vi "Ad-Hoc.vi"(7 "Minutes to wait":u32, 8 "error in":errorcluster, 11 "Ad-Hoc Installers":T1 {"MachineName" items=["Machine-06", "Machine-01", "Machine-02", "Machine-03", "Machine-04"]}) -> (0 "error Out":errorcluster, 3 "Array":path[](array[path]))   [LabVIEW 2013]
uses:
  MachineNames.ctl
  ControlAd-Hoc.ctl
  <vilib>/Utility/config.llb/Read Key (String).vi
  <vilib>/Utility/config.llb/NI_LVConfig.lvlib
panel:
  out "Ring 2":T2=3 items=["Machine-01", "Machine-02", "Machine-03", "Machine-04"]
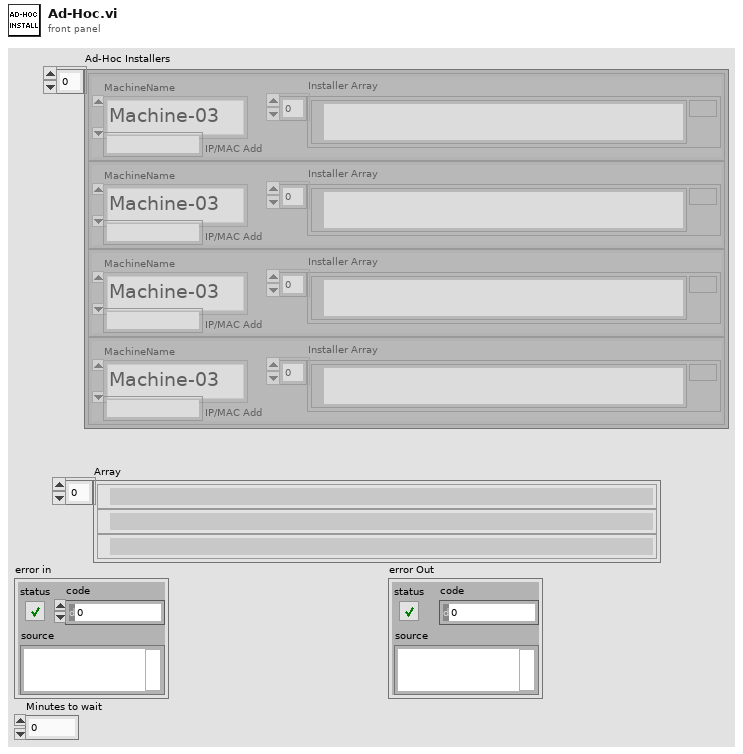
[diagram p1: front panel]
types:
  T1 = typedef "ControlAd-Hoc.ctl" = cluster{"Installer Array":path[], "MachineName":T2, "IP/MAC Add":string}[]
  T2 = typedef "MachineNames.ctl" = u16
  T3 = typedef "NI_LVConfig.lvlib/Config Data RefNum.ctl" = refnum<k1>
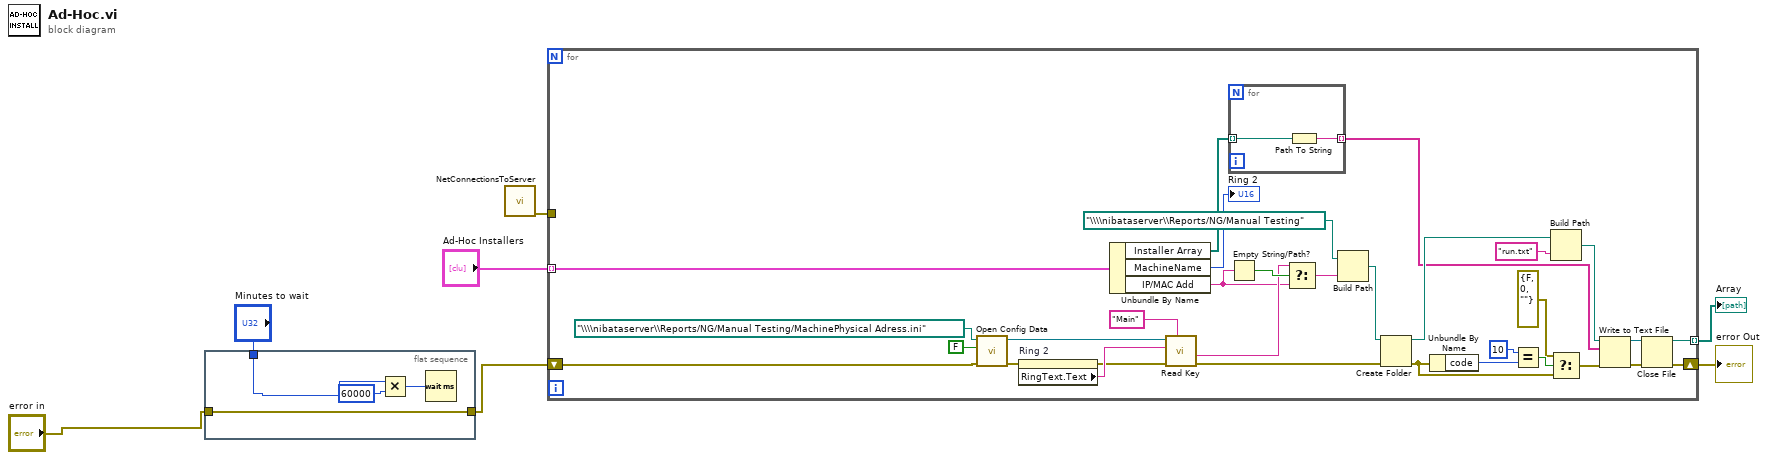
[diagram p0: block diagram]
diagram:
  n1 = flat-sequence {
    tunnel: "error in" -> [w11]
    tunnel: [w11] -> w2
    tunnel: "Minutes to wait" -> [w8]
    frame #0 {
      n2 = Multiply(x=w8, y=u32 60000) -> (x*y=w10:u32)
      n3 = Wait (ms)(milliseconds to wait=w10) -> ()  [unwired: 1 out]
    }
  }
  n4 = call "NetConnectionsToServer.vi"() -> ("error out"=w4:errorcluster)  [unwired: 11 in]
  n5 = for {
    tunnel: "Ad-Hoc Installers" -> [w43] mode=indexing
    tunnel: [w35] -> w7 mode=indexing
    shift-right: [w25] -> w5
    shift-left: w2 -> [w24]
    tunnel: w4 -> [_]
    n6 = call <vilib>:"Open Config Data.vi"("error in (no error)"=w24, "create file if necessary (T)"=FALSE, "configuration file path"=path "\\\\nibataserver\\Reports/NG/Manual Testing/MachinePhysical Adress.ini") -> ("error out"=w27:errorcluster, "refnum"=w31:T3)  [unwired: 6 in, 1 out]
    n7 = property on="Ring 2" class="Ring (strict)"(error in=w27) -> (error out=w28:errorcluster, "RingText.Text"=w29:string)  [unwired: 1 in, 1 out]
    n8 = Unbundle By Name(w43) -> ("Installer Array"=w42:path[], "MachineName"=→"Ring 2":T2, "IP/MAC Add"=w13:string)
    n9 = call-poly <vilib>:"Read Key.vi"("section"="Main", "error in (no error)"=w28, "key"=w29, "refnum"=w31) -> ("error out"=w16:errorcluster, "value"=w14:string)  [unwired: 4 in, 2 out]
    n10 = for {
      tunnel: w42 -> [w45] mode=indexing
      tunnel: [w44] -> w34 mode=indexing
      n11 = Path To String(path=w45) -> (string=w44:string)
    }
    n12 = Empty String/Path?(string/path=w13) -> (empty?=w15:bool)
    n13 = Select(t=w14, s=w15, f=w13) -> (s? t:f=w12:string)
    n14 = Build Path(base path=path "\\\\nibataserver\\Reports/NG/Manual Testing", name or relative path=w12) -> (appended path=w38:path)
    n15 = Create Folder(path (use dialog)=w38, error in=w16) -> (created path=w37:path, error out=w19:errorcluster)  [unwired: 1 in, 1 out]
    n16 = Unbundle By Name(w19) -> ("code"=w23:i32)
    n17 = Equal?(x=10, y=w23) -> (x = y?=w21:bool)
    n18 = Build Path(base path=w37, name or relative path="run.txt") -> (appended path=w40:path)
    n19 = Select(t=errorcluster {"status"=FALSE, "code"=0, "source"=""} ("error constant"), s=w21, f=w19) -> (s? t:f=w18:errorcluster)
    n20 = Write to Text File(file (use dialog)=w40, text=w34, error in=w18) -> (refnum out=w36:refnum<file>, error out=w26:errorcluster)  [unwired: 1 in, 1 out]
    n21 = Close File(refnum=w36, error in=w26) -> (path=w35:path, error out=w25:errorcluster)
  }
  "Array" <- w7
  "error Out" <- w5
